vi "Main2.vi"() -> ()   [LabVIEW 2014]
doc: "This sample project is built upon the standard state machine template and shows how you could create an application that acquires, analyzes, and presents data. It includes functionality for presenting configuration dialogs, preserving settings between executions, loading and saving data, as well as exporting graph images and text files.\n\nIt is most appropriate for data that is acquired instantly as it does not allow for screen updates mid acquisition nor does it allow for continuous streaming to disk."
uses:
  controls/DAQSettings.ctl
  controls/TriggerMode.ctl
  controls/AspicSettings.ctl
  controls/AspicMode.ctl
  controls/Timeslice.ctl
  controls/SystemSet.ctl
  common/Comm/path.ctl
  controls/Data OK.ctl
  controls/Data.ctl
  controls/UI References.ctl
  controls/Graph Data.ctl
  <vilib>/Utility/miscctls.llb/LVAnnotationListTypeDef.ctl
  <vilib>/Utility/miscctls.llb/LVCursorListTypeDef.ctl
  controls/User Specified Data.ctl
  controls/HW Configuration.ctl
  controls/Simulated Signal Type.ctl
  controls/Analysis Configuration.ctl
  controls/New Data Behavior.ctl
  controls/Network.ctl
  controls/CommSelect.ctl
  common/Comm/analysis.ctl
  controls/State.ctl
  global/Global ADCarray.vi
panel:
  out "End acq":u32
  out "Begin acq":u32
  out "Path":T1={"TS file"=path "C:/Users/lpnhe/Desktop/Labview/damic/DAMIC-LTC/DamicLTC-seul-Essai.txt", "Log file"=path "C:/DAMIC/DAMIC-LTC/Data/log.txt", "Log Directory"=path "C:/DAMIC/DAMIC-LTC/Data", "Output aspic file folder"=path "C:/Users/lpnhe/Desktop/Labview/damic/DAMIC-LTC/Data", "TSfile folder"=path "C:/Users/lpnhe/Desktop/Labview/damic/DAMIC_TIMESLICE"}
  out "size(s)":i32[](array[numeric])
  in  "Curve fitting":bool
  in  "Load  Config":bool
  in  "Save  Config":bool
  in  "Path Settings":bool
  out "System Set":T2
  in  "SystemSet":bool
  in  "DAQSettings":bool
  in  "Timeslice":bool
  in  "Network Settings":bool
  in  "ASPIC Settings":bool
  in  "Snapshot":bool
  in  "Analyze":bool
  in  "Clear":bool
  in  "Exit":bool
  in  "Acquire":bool
  in  "Export":bool
  in  "Save Graph":bool
  in  "Load Graph":bool
  out "Data OK":T3
  in  "Tab Control":enum32{"Data", "Fitting", "FFT", "Results"}(tab)
  out "Time needed(s)":u32
  out "Graph":waveform(dbl)[](graph)
  in  "Display":bool
  in  "Channel":T4(ring)
  out "Results":T5
  out "timeslice":T6
  out "Aspic Seeting":T7 {"RC" format="%b"; "Gain" format="%b"}
  out "DAQ Settings":T9
  out "Status Bar":string
  # "CH0"
  # "CH1"
  # "CH2"
  # "CH3"
  # "CH4"
  # "CH5"
  # "CH6"
  # "CH7"
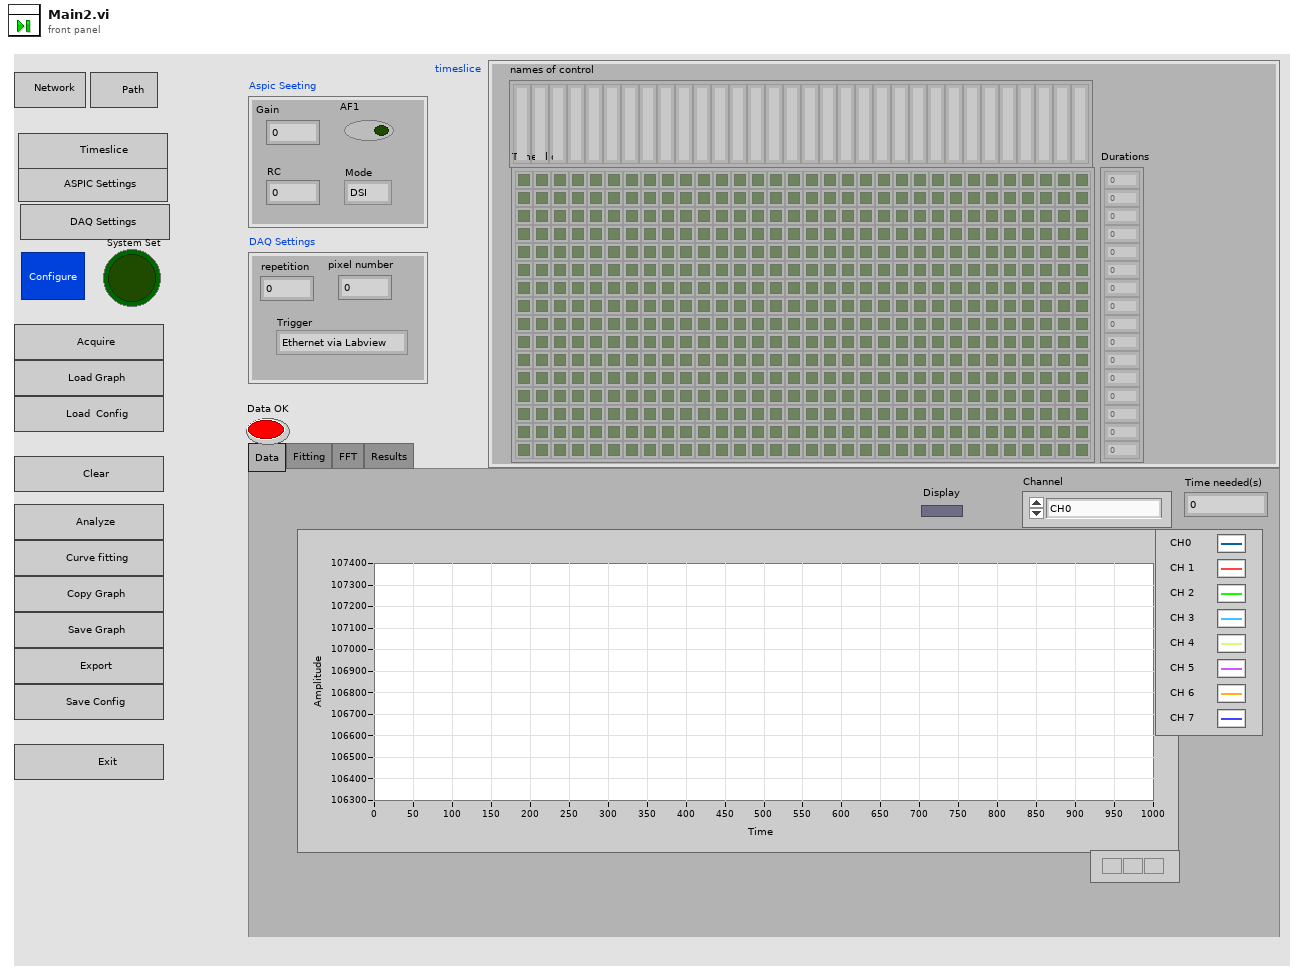
[diagram p1: front panel]
types:
  T1 = typedef "path.ctl" = cluster{"TS file":path, "Log file":path, "Log Directory":path, "Output aspic file folder":path, "TSfile folder":path}
  T2 = typedef "SystemSet.ctl" = bool
  T3 = typedef "Data OK.ctl" = bool
  T4 = enum16{"CH0", "CH1", "CH2", "CH3", "CH4", "CH5", "CH6", "CH7", "All (TDMS)"}
  T5 = cluster{"Max":i32[], "Min":i32[], "Average":dbl[], "S.D":dbl[], "Variance":dbl[]}
  T6 = typedef "Timeslice.ctl" = cluster{"Time slice":bool[][], "Durations":dbl[], "names of control":string[]}
  T7 = typedef "AspicSettings.ctl" = cluster{"Gain":u8, "RC":u8, "aspic1Data":u32[], "aspic2Data":u32[], "AF1":bool, "Mode":T8}
  T8 = typedef "AspicMode.ctl" = enum16{"DSI", "TM"}
  T9 = typedef "DAQSettings.ctl" = cluster{"pixel number":u32, "repetition":u32, "Trigger":T10}
  T10 = typedef "TriggerMode.ctl" = enum16{"Ethernet via Labview", "SMA (1.8V)"}
  T11 = typedef "State.ctl" = enum16{"Initialize", "Wait for Event", "Update UI", "Network", "Path", "Configure", "DAQSettings", "Timeslice", "Set Sytem", "Acquire", "Load Data", "Save Data", "Load config", "Save config", "Clear Data", "Export Data", "Analyze", "Curve fitting", "Copy Graph", "Exit"}
  T12 = typedef "Data.ctl" = cluster{"UI References":T13, "Graph Data":T14, "User Specified":T17, "System Set":T2, "Results":T24, "Data OK":T3}
  T13 = typedef "UI References.ctl" = cluster{"Exit Ref":refnum<vi>, "Save Ref":refnum<vi>, "Open Ref":refnum<vi>, "Export Ref":refnum<vi>, "Acquire Ref":refnum<vi>, "Configure Ref":refnum<vi>, "Graph Ref":refnum<vi>, "Clear Ref":refnum<vi>, "Analyze Ref":refnum<vi>, "Status Ref":refnum<vi>, "Snapshot Ref":refnum<vi>, "Network Ref":refnum<vi>, "Timeslice Ref":refnum<vi>, "DAQSetting Ref":refnum<vi>, "SystemSet":refnum<vi>, "Path ref":refnum<vi>, "Data OK Ref":refnum<vi>}
  T14 = typedef "Graph Data.ctl" = cluster{"Data":waveform(dbl)[], "Annotation List":T15, "Cursor List":T16, "Analysis Data":waveform(dbl)[]}
  T15 = typedef "LVAnnotationListTypeDef.ctl" = cluster{"Name":string, "Color":u32, "Style":u8, "Point Style":u8, "Name Visible":bool, "Allow Drag":bool, "Annotation Mode":u32, "Plot":i32, "Index":i32, "Position":cluster{"X":dbl, "Y":dbl}, "X Scale":u32, "Y Scale":u32, "Show Arrow":bool, "Lock Name":bool, "Plot Area":i32, "Label Offset":cluster{"X":dbl, "Y":dbl}}[]
  T16 = typedef "LVCursorListTypeDef.ctl" = cluster{"Name":string, "Color":u32, "Style":u8, "Point Style":u8, "Name Visible":bool, "Allow Drag":bool, "Cursor Mode":u32, "Plot":i32, "Index":i32, "Position":cluster{"X":dbl, "Y":dbl}, "X Scale":u32, "Y Scale":u32, "Watch Plots":i32[], "Watch All Plots":bool, "Plot Area":i32, "Label Offset":cluster{"X":dbl, "Y":dbl}}[]
  T17 = typedef "User Specified Data.ctl" = cluster{"Hardware Configuration":T18, "Analysis Configuration":T20, "New Data Behavior":T21, "Aspic Seeting":T7, "Network":T22, "timeslice":T6, "Acquisition Settings":T9, "CommSelect":T23, "Path":T1}
  T18 = typedef "HW Configuration.ctl" = cluster{"HW Refnum <Replace Me>":string, "Signal Type <Replace Me>":T19}
  T19 = typedef "Simulated Signal Type.ctl" = enum16{"Sine Wave", "Square Wave"}
  T20 = typedef "Analysis Configuration.ctl" = cluster{"Statistics":bool}
  T21 = typedef "New Data Behavior.ctl" = enum16{"Replace", "Overlay", "Append"}
  T22 = typedef "Network.ctl" = cluster{"invert_send":bool, "Number of datagrams to read":u32, "max bytes/read":i32, "Timeout":i32, "host":string, "Port Receive":u16}
  T23 = typedef "CommSelect.ctl" = enum16{"startTSL", "writeCABAC", "readCABAC", "resetCABAC", "emissionTest", "regRead", "executeASPIC", "resetASPIC", "resetFifo18ASPIC", "resetFifo16ASPIC", "LabviewDamicStart"}
  T24 = typedef "analysis.ctl" = cluster{"Max":i32[], "Min":i32[], "Average":dbl[], "S.D":dbl[], "Variance":dbl[]}
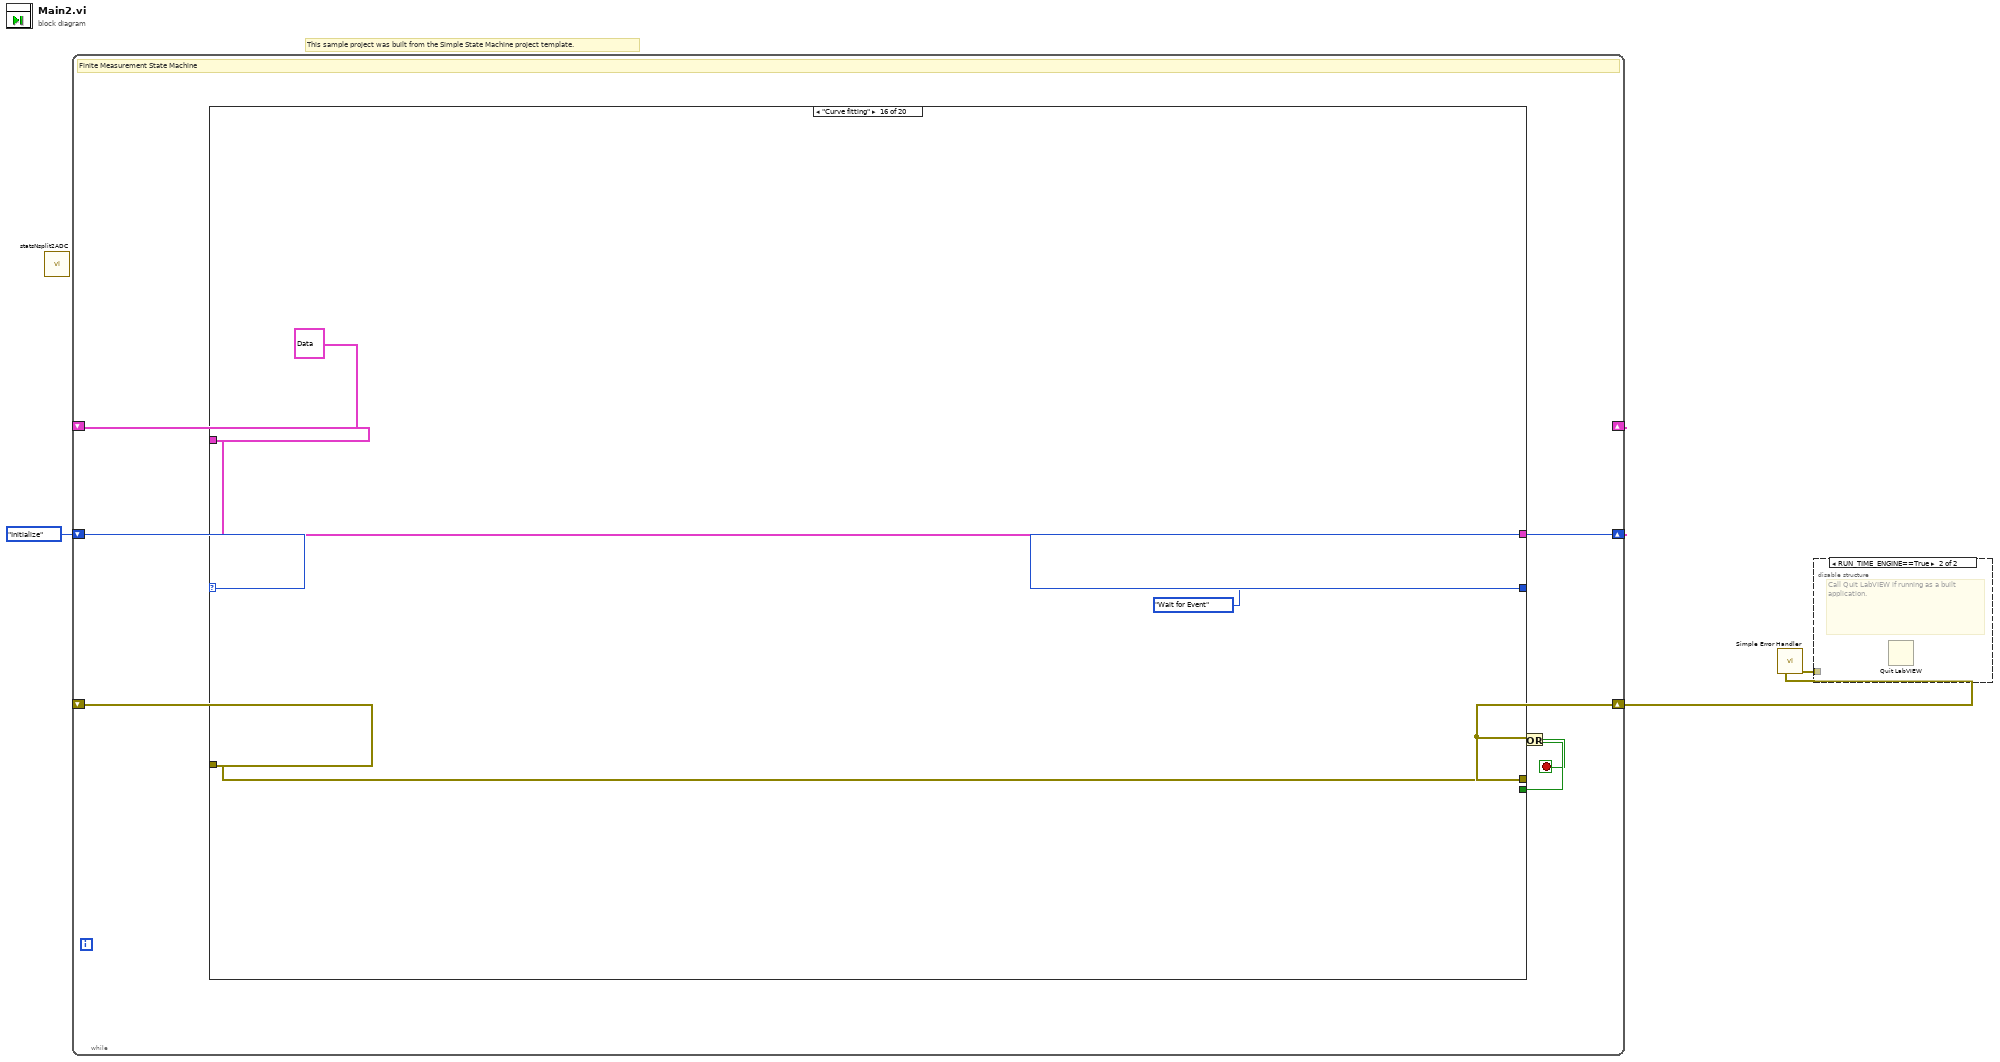
[diagram p0: block diagram]
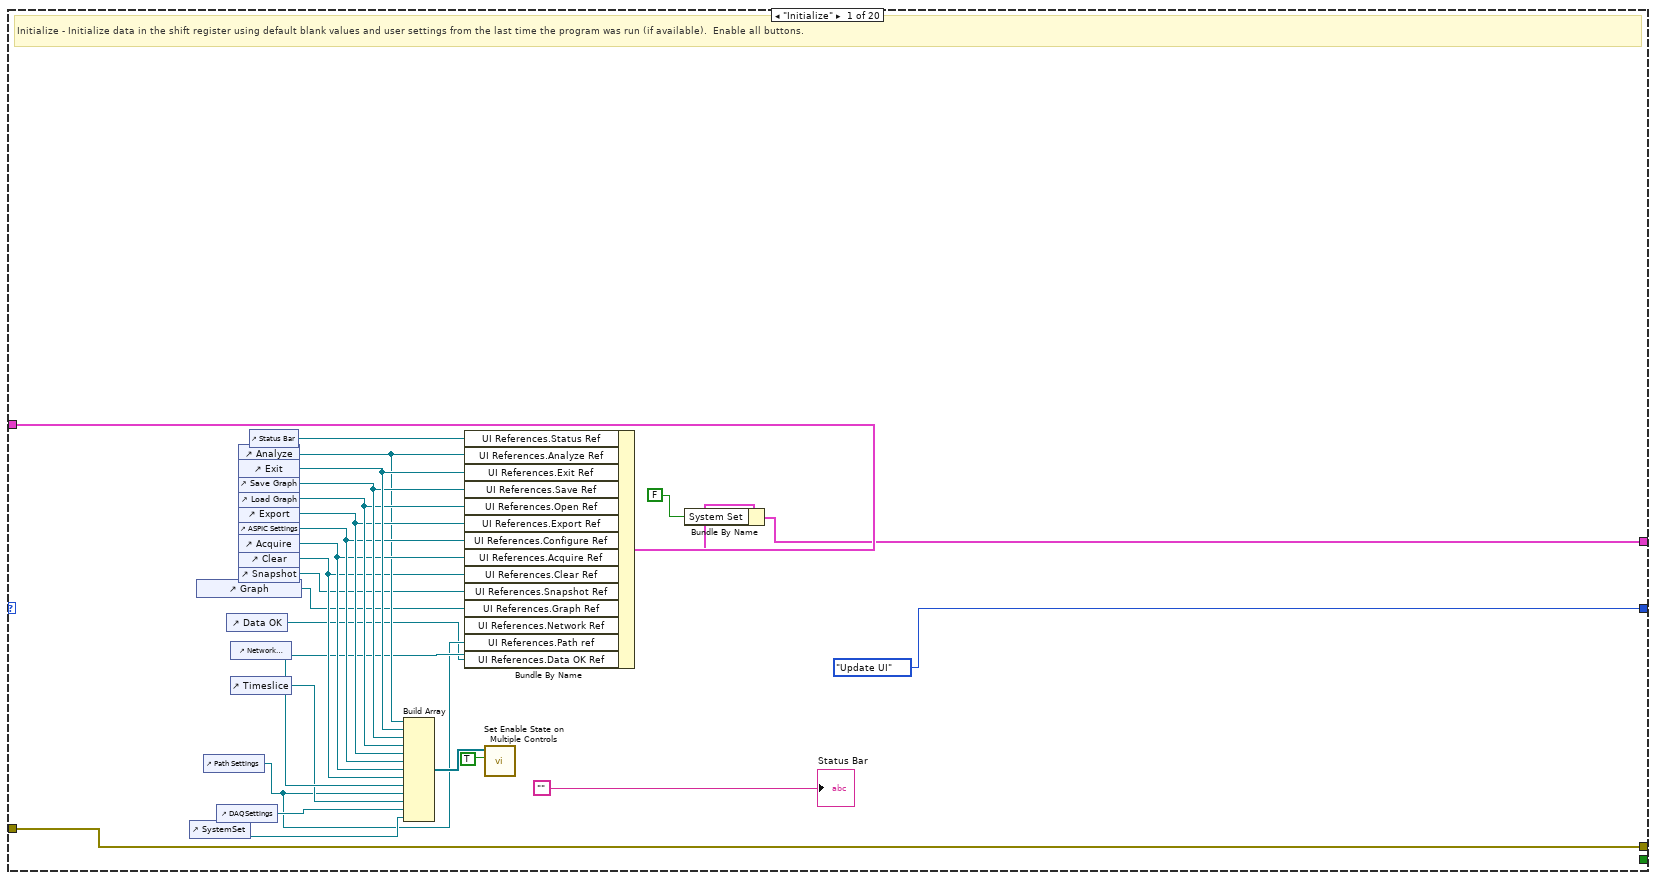
[diagram p3: hidden frame]
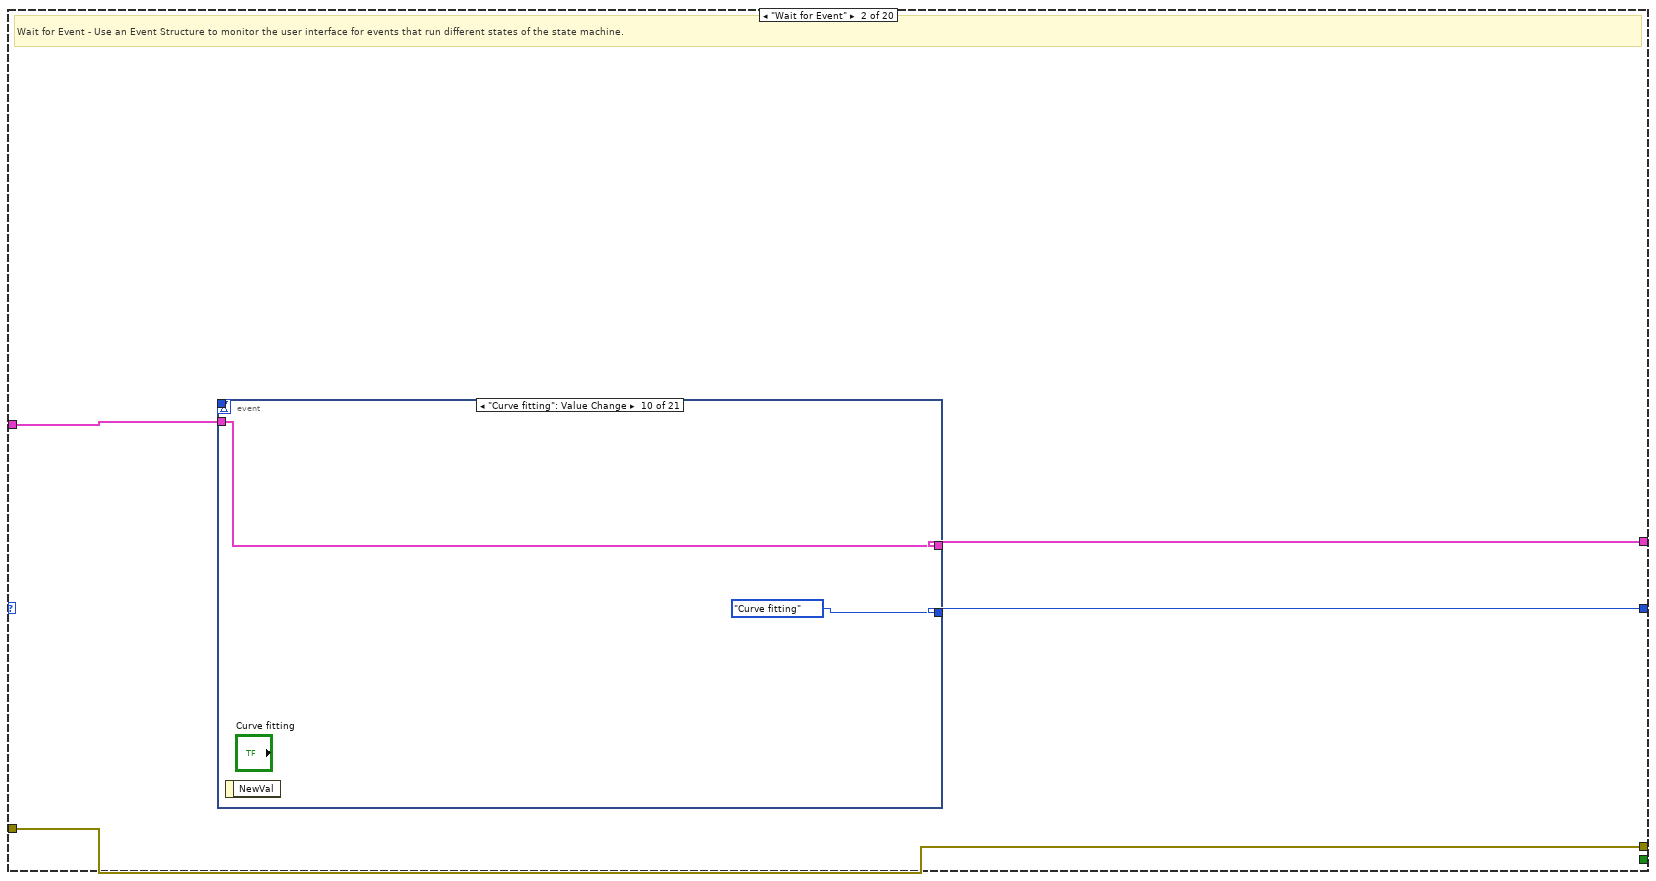
[diagram p4: hidden frame]
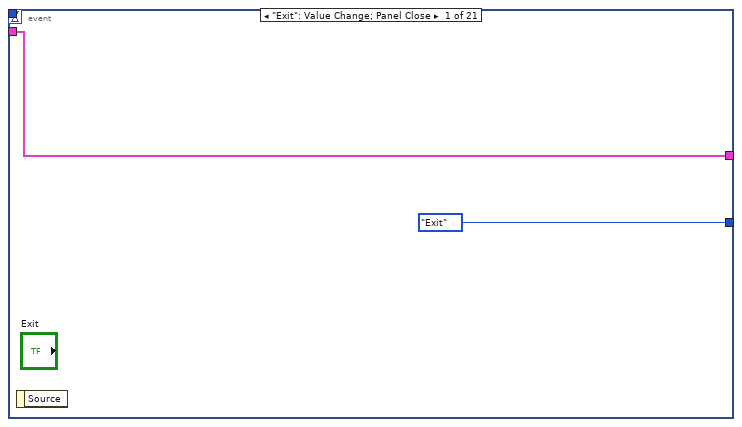
[diagram p5: hidden frame]
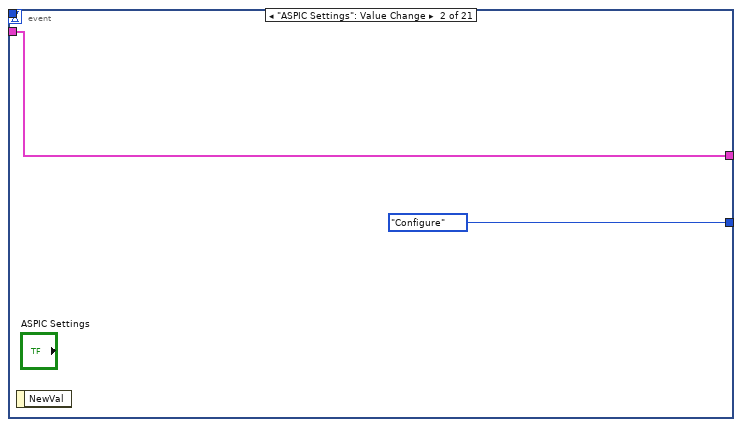
[diagram p6: hidden frame]
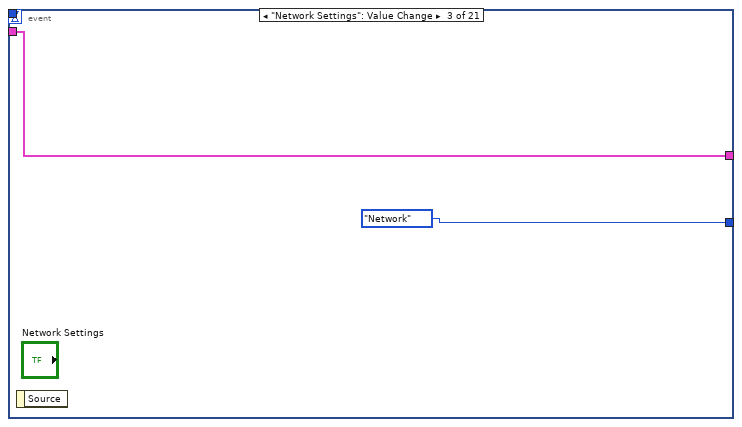
[diagram p7: hidden frame]
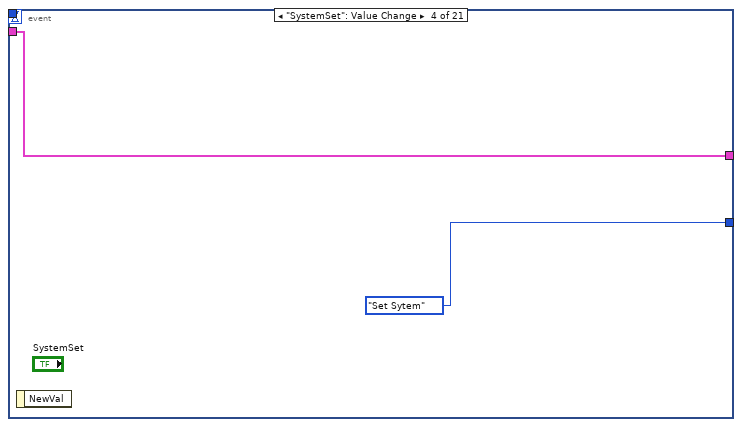
[diagram p8: hidden frame]
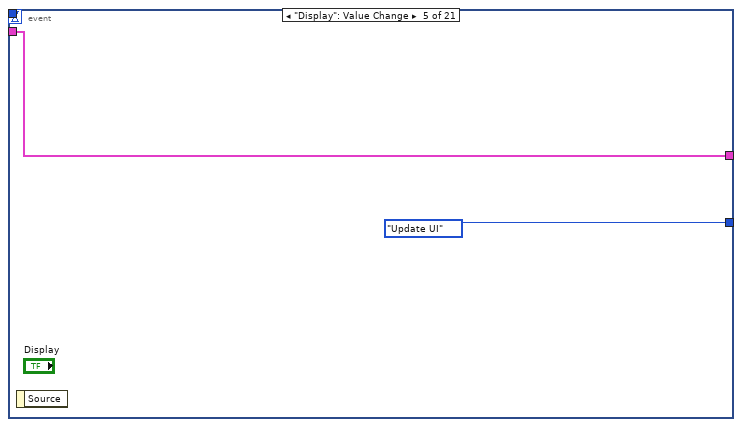
[diagram p9: hidden frame]
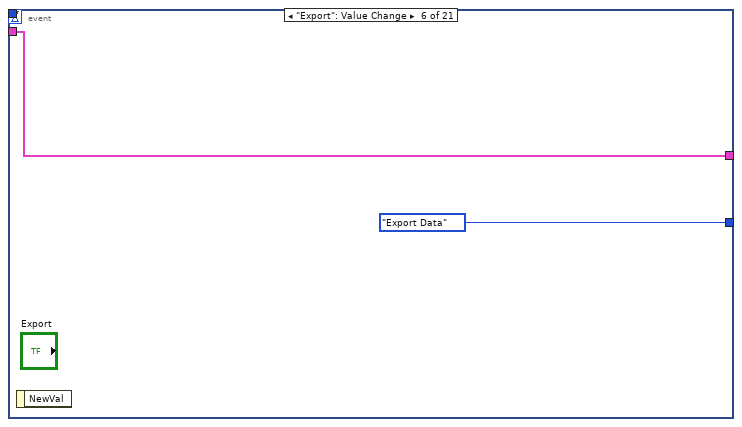
[diagram p10: hidden frame]
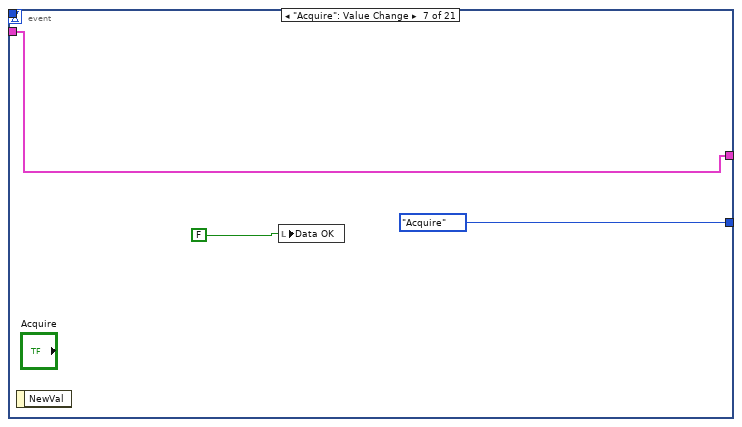
[diagram p11: hidden frame]
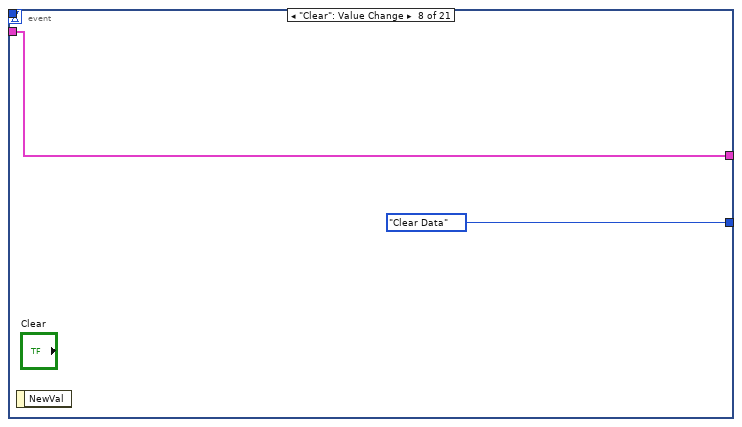
[diagram p12: hidden frame]
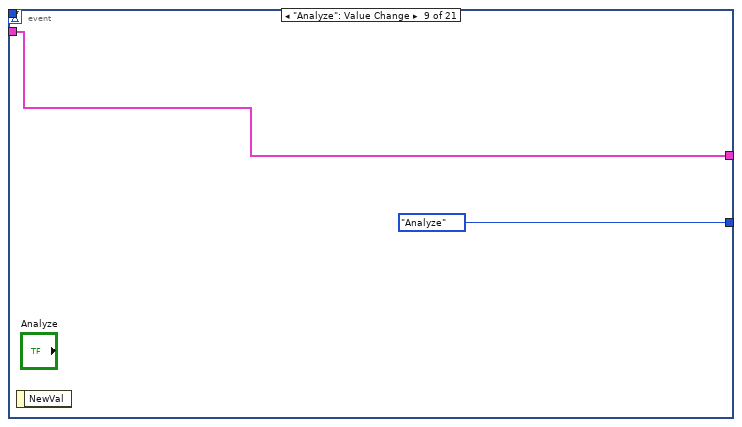
[diagram p13: hidden frame]
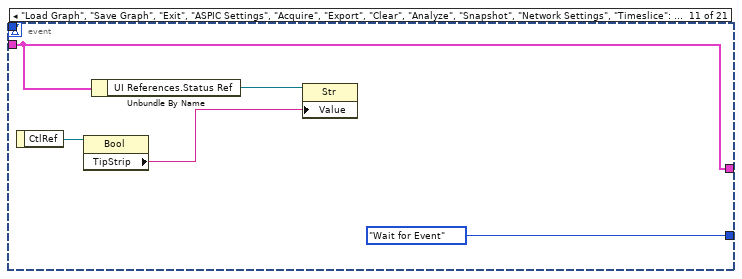
[diagram p14: hidden frame]
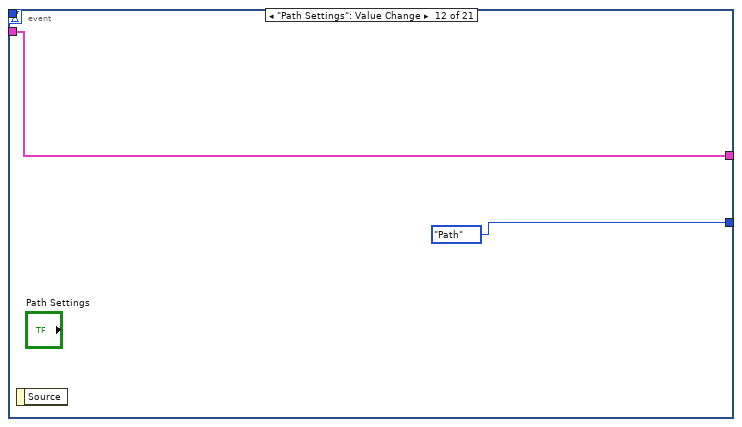
[diagram p15: hidden frame]
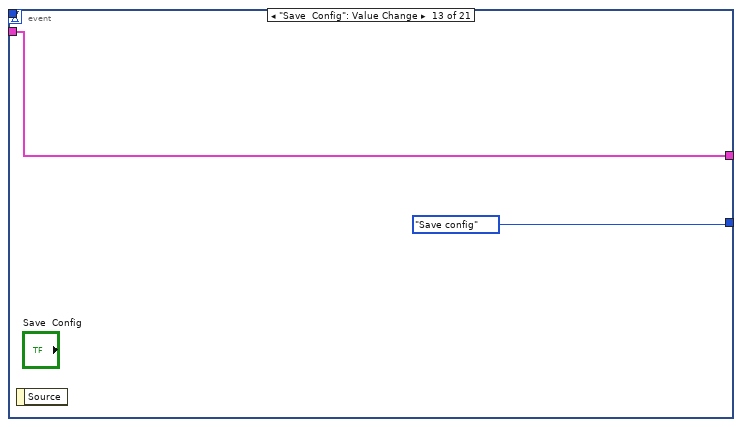
[diagram p16: hidden frame]
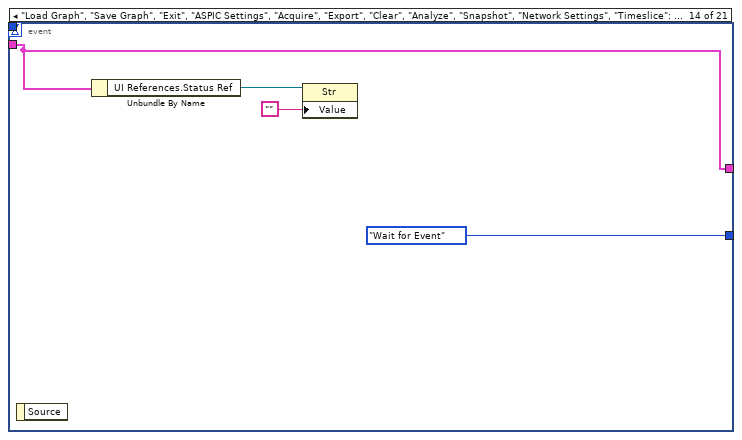
[diagram p17: hidden frame]
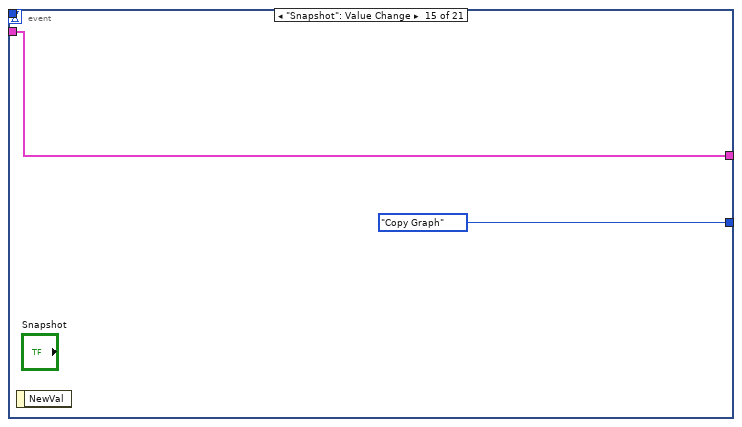
[diagram p18: hidden frame]
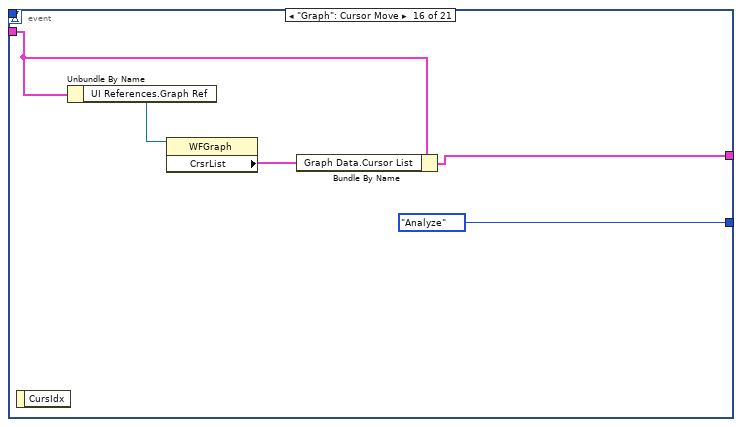
[diagram p19: hidden frame]
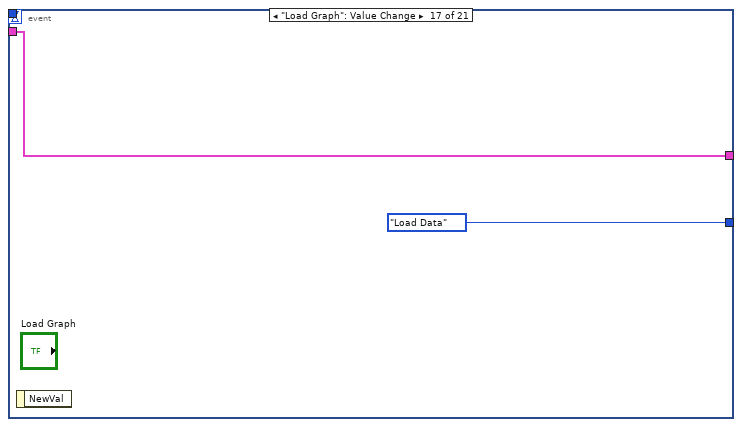
[diagram p20: hidden frame]
diagram:
  # "This sample project was built from the Simple State Machine project template."
  n1 = call "statsNsplit2ADC.vi"() -> ()  [unwired: 4 in, 4 out]
  n2 = while {
    shift-right: [w11] -> _
    shift-left: State."Initialize" ("Next State") -> [w12]
    shift-right: [w5] -> w4
    shift-left: _ -> [w6]
    shift-right: [w7] -> _
    shift-left: T12 {"UI References"={"Exit Ref"=refnum, "Save Ref"=refnum, "Open Ref"=refnum, "Export Ref"=refnum, "Acquire Ref"=refnum, "Configure Ref"=refnum, "Graph Ref"=refnum, "Clear Ref"=refnum, "Analyze Ref"=refnum, "Status Ref"=refnum, "Snapshot Ref"=refnum, "Network Ref"=refnum, "Timeslice Ref"=refnum, "DAQSetting Ref"=refnum, "SystemSet"=refnum, "Path ref"=refnum, "Data OK Ref"=refnum}, "Graph Data"={"Data"=[], "Annotation List"=[], "Cursor List"=[], "Analysis Data"=[]}, "User Specified"={"Hardware Configuration"={"HW Refnum <Replace Me>"="", "Signal Type <Replace Me>"=enum."Sine Wave"}, "Analysis Configuration"={"Statistics"=TRUE}, "New Data Behavior"=enum."Replace", "Aspic Seeting"={"Gain"=0, "RC"=0, "aspic1Data"=[], "aspic2Data"=[], "AF1"=FALSE, "Mode"=enum."TM"}, "Network"={"invert_send"=TRUE, "Number of datagrams to read"=5000, "max bytes/read"=2500, "Timeout"=4000, "host"="192.168.1.18", "Port Receive"=5678}, "timeslice"={"Time slice"=[], "Durations"=[], "names of control"=[]}, "Acquisition Settings"={"pixel number"=0, "repetition"=0, "Trigger"=enum."Ethernet via Labview"}, "CommSelect"=enum."resetFifo18ASPIC", "Path"={"TS file"=path "C:/Users/lpnhe/Desktop/Labview/damic/DAMIC-LTC/DamicLTC-seul-Essai.txt", "Log file"=path "C:/DAMIC/DAMIC-LTC/Data/log.txt", "Log Directory"=path "C:/DAMIC/DAMIC-LTC/Data", "Output aspic file folder"=path "C:/Users/lpnhe/Desktop/Labview/damic/DAMIC-LTC/Data", "TSfile folder"=path "C:/Users/lpnhe/Desktop/Labview/damic/DAMIC_TIMESLICE"}}, "System Set"=FALSE, "Results"={"Max"=[], "Min"=[], "Average"=[], "S.D"=[], "Variance"=[]}, "Data OK"=FALSE} ("Data") -> [w8]
    stop <- w9 stop-if-true
    # "Finite Measurement State Machine"
    n3 = case shown="\"Curve fitting\"" w12 {
      tunnel: [State."Update UI" ("Next State") w42 State."Wait for Event" ("(Value Not Used)") State."Update UI" ("Next State if true") w154 State."Update UI" ("Next State if true") State."Update UI" ("Next State if true") w184 State."Update UI" ("States") w230 State."Update UI" ("(Value Not Used)") State."Wait for Event" ("(Value Not Used)") State."Wait for Event" ("(Value Not Used)") State."Update UI" ("(Value Not Used)") State."Update UI" ("(Value Not Used)") State."Wait for Event" ("Next State") State."Wait for Event" ("(Value Not Used)") w338 State."Update UI" ("Next State") State."Wait for Event" ("Next State")] -> w11
      tunnel: [_ _ _ _ _ _ _ _ _ _ _ _ _ _ _ _ _ w337 _ _] -> w10
      tunnel: w8 -> [w17 w41 w105 w144 w155 w166 w173 w182 w198 w229 w276 w292 w305 w318 w323 w329 w333 w336 w344 w349]
      tunnel: [w14 w40 w105 w138 w146 w158 w167 w176 w194 w226 w275 w292 w305 w317 w321 w329 w333 w336 w343 w349] -> w7
      tunnel: w6 -> [w22 w39 w106 w142 w152 w165 w172 w188 w196 w228 w273 w291 w304 w316 w325 w328 w332 w335 w341 w351]
      tunnel: [w22 w39 w106 w141 w151 w162 w171 w188 w189 w227 w272 w290 w303 w316 w324 w328 w331 w335 w340 w350] -> w5
      frame "Initialize" {
        # "Initialize - Initialize data in the shift register using default blank values and user settings from the last time the program was run (if available).  Enable all buttons."
        n4 = control-ref of="SystemSet"() -> (w19:refnum<vi>)
        n5 = control-ref of="Graph"() -> (w24:refnum<vi>)
        n6 = control-ref of="Path Settings"() -> (w18:refnum<vi>)
        n7 = control-ref of="DAQSettings"() -> (w20:refnum<vi>)
        n8 = control-ref of="Data OK"() -> (w13:refnum<vi>)
        n9 = control-ref of="Network Settings"() -> (w23:refnum<vi>)
        n10 = control-ref of="Timeslice"() -> (w21:refnum<vi>)
        n11 = control-ref of="Analyze"() -> (w30:refnum<vi>)
        n12 = control-ref of="Exit"() -> (w37:refnum<vi>)
        n13 = control-ref of="Save Graph"() -> (w36:refnum<vi>)
        n14 = control-ref of="Load Graph"() -> (w35:refnum<vi>)
        n15 = control-ref of="Export"() -> (w34:refnum<vi>)
        n16 = control-ref of="ASPIC Settings"() -> (w33:refnum<vi>)
        n17 = control-ref of="Acquire"() -> (w32:refnum<vi>)
        n18 = control-ref of="Clear"() -> (w28:refnum<vi>)
        n19 = control-ref of="Snapshot"() -> (w25:refnum<vi>)
        n20 = control-ref of="Status Bar"() -> (w29:refnum<vi>)
        n21 = Build Array(w30, w37, w36, w35, w34, w33, w32, w28, w23, w18, w21, w20, w19) -> (w31:refnum<vi>[])
        n22 = Bundle By Name(cluster=w17, "UI References.Status Ref"=w29, "UI References.Analyze Ref"=w30, "UI References.Exit Ref"=w37, "UI References.Save Ref"=w36, "UI References.Open Ref"=w35, "UI References.Export Ref"=w34, "UI References.Configure Ref"=w33, "UI References.Acquire Ref"=w32, "UI References.Clear Ref"=w28, "UI References.Snapshot Ref"=w25, "UI References.Graph Ref"=w24, "UI References.Network Ref"=w23, "UI References.Path ref"=w18, "UI References.Data OK Ref"=w13) -> (w16:T12)
        n23 = call "Set Enable State on Multiple Controls.vi"("Enable?"=TRUE, "Controls"=w31) -> ()  [unwired: 10 in]
        n24 = Bundle By Name(cluster=w16, "System Set"=FALSE) -> (w14:T12)
        "Status Bar" <- "" ("Status Bar")
      }
      frame "Wait for Event" {
        # "Wait for Event - Use an Event Structure to monitor the user interface for events that run different states of the state machine."
        n25 = event shown="[9] \"Curve fitting\": Value Change" {
          selector: _ -> [_ _ _ _ _ _ _ _ _ _ _ _ _ _ _ _ _ _ _ _ _]
          dyn-events: _ -> [_ _ _ _ _ _ _ _ _ _ _ _ _ _ _ _ _ _ _ _ _]
          timeout: _ -> [_ w46 _ _ _ _ _ _ _ _ _ _ _ _ _ _ _ _ _ _ _]
          tunnel: [State."Exit" ("Next State") State."Configure" ("Next State") State."Network" ("States") State."Set Sytem" ("States") State."Update UI" ("States") State."Export Data" ("Next State") State."Acquire" ("Next State") State."Clear Data" ("Next State") State."Analyze" ("Next State") State."Curve fitting" ("Next State") State."Wait for Event" ("Next State") State."Path" ("Next State") State."Save config" ("Next State") State."Wait for Event" ("Next State") State."Copy Graph" ("Next State") State."Analyze" ("Next State") State."Load Data" ("Next State") State."Save Data" ("Next State") State."Load config" ("Next State") State."Timeslice" ("States") State."DAQSettings" ("States")] -> w42
          tunnel: [_ w46 _ _ _ _ _ _ _ _ _ _ _ _ _ _ _ _ _ _ _] -> _
          tunnel: w41 -> [w43 w45 w49 w51 w53 w54 w57 w59 w61 w64 w65 w71 w73 w74 w78 w81 w85 w87 w90 w92 w94]
          tunnel: [w43 w45 w49 w51 w53 w54 w57 w59 w61 w64 w65 w71 w73 w74 w78 w80 w85 w87 w90 w92 w94] -> w40
          event "Exit": Value Change; Panel Close {
            n26 = event-data() -> ()  [unwired: 1 in, 1 out]
          }
          event "ASPIC Settings": Value Change {
            n27 = event-data() -> ()  [unwired: 1 in, 1 out]
          }
          event "Network Settings": Value Change {
            n28 = event-data() -> ()  [unwired: 1 in, 1 out]
          }
          event "SystemSet": Value Change {
            n29 = event-data() -> ()  [unwired: 1 in, 1 out]
          }
          event "Display": Value Change {
            n30 = event-data() -> ()  [unwired: 1 in, 1 out]
          }
          event "Export": Value Change {
            n31 = event-data() -> ()  [unwired: 1 in, 1 out]
          }
          event "Acquire": Value Change {
            n32 = event-data() -> ()  [unwired: 1 in, 1 out]
            n33 = local write "Data OK"(FALSE) -> ()
          }
          event "Clear": Value Change {
            n34 = event-data() -> ()  [unwired: 1 in, 1 out]
          }
          event "Analyze": Value Change {
            n35 = event-data() -> ()  [unwired: 1 in, 1 out]
          }
          event "Curve fitting": Value Change {
            n36 = event-data() -> ()  [unwired: 1 in, 1 out]
          }
          event "Load Graph", "Save Graph", "Exit", "ASPIC Settings", "Acquire", "Export", "Clear", "Analyze", "Snapshot", "Network Settings", "Timeslice": Mouse Enter {
            n37 = event-data() -> ("CtlRef"=w69:refnum<vi>)  [unwired: 1 in]
            n38 = property class="Bool"(reference=w69) -> ("TipStrip"=w67:string)  [unwired: 1 in, 2 out]
            n39 = Unbundle By Name(w65) -> ("UI References.Status Ref"=w68:refnum<vi>)
            n40 = property class="Str"(reference=w68, "Value"=w67) -> ()  [unwired: 1 in, 2 out]
          }
          event "Path Settings": Value Change {
            n41 = event-data() -> ()  [unwired: 1 in, 1 out]
          }
          event "Save  Config": Value Change {
            n42 = event-data() -> ()  [unwired: 1 in, 1 out]
          }
          event "Load Graph", "Save Graph", "Exit", "ASPIC Settings", "Acquire", "Export", "Clear", "Analyze", "Snapshot", "Network Settings", "Timeslice": Mouse Leave {
            n43 = event-data() -> ()  [unwired: 1 in, 1 out]
            n44 = Unbundle By Name(w74) -> ("UI References.Status Ref"=w77:refnum<vi>)
            n45 = property class="Str"(reference=w77, "Value"="") -> ()  [unwired: 1 in, 2 out]
          }
          event "Snapshot": Value Change {
            n46 = event-data() -> ()  [unwired: 1 in, 1 out]
          }
          event "Graph": Cursor Move {
            n47 = event-data() -> ()  [unwired: 1 in, 1 out]
            n48 = Unbundle By Name(w81) -> ("UI References.Graph Ref"=w83:refnum<vi>)
            n49 = property class="WFGraph"(reference=w83) -> ("CrsrList"=w82:T16)  [unwired: 1 in, 2 out]
            n50 = Bundle By Name(cluster=w81, "Graph Data.Cursor List"=w82) -> (w80:T12)
          }
          event "Load Graph": Value Change {
            n51 = event-data() -> ()  [unwired: 1 in, 1 out]
          }
          event "Save Graph": Value Change {
            n52 = event-data() -> ()  [unwired: 1 in, 1 out]
          }
          event "Load  Config": Value Change {
            n53 = event-data() -> ()  [unwired: 1 in, 1 out]
          }
          event "Timeslice": Value Change {
            n54 = event-data() -> ()  [unwired: 1 in, 1 out]
          }
          event "DAQSettings": Value Change {
            n55 = event-data() -> ()  [unwired: 1 in, 1 out]
          }
        }
      }
      frame "Update UI" {
        # "These buttons should be disabled when there is no data visible."
        # "Update UI - Update the graph using the waveform data stored in the shift register.  If there is no data to display disable buttons that act on the current data."
        n56 = Unbundle By Name(w105) -> ("Results"=→"Results":T24, "Graph Data.Data"=w99:waveform(dbl)[], "Graph Data.Annotation List"=w109:T15, "Graph Data.Cursor List"=w108:T16)
        n57 = Unbundle By Name(w105) -> ("User Specified.Path"=→"Path":T1, "User Specified.timeslice"=→"timeslice":T6, "User Specified.Aspic Seeting"=→"Aspic Seeting":T7, "User Specified.Acquisition Settings"=→"DAQ Settings":T9, "System Set"=→"System Set":T2, "Data OK"=→"Data OK":T3)
        n58 = Unbundle By Name(w105) -> ("UI References.Clear Ref"=w115:refnum<vi>, "UI References.Analyze Ref"=w114:refnum<vi>, "UI References.Save Ref"=w118:refnum<vi>, "UI References.Export Ref"=w112:refnum<vi>, "UI References.Snapshot Ref"=w113:refnum<vi>)
        n59 = case shown="\"All (TDMS)\"" "Channel" {
          tunnel: w99 -> [w121 w123 w125 w127 w129 w131 w133 w135 w136]
          tunnel: [w120 w122 w124 w126 w128 w130 w132 w134 w136] -> w98
          frame "CH0", Default {
            n60 = Decimate 1D Array(w121) -> (w120:waveform(dbl)[])  [unwired: 7 out]
          }
          frame "CH1" {
            n61 = Decimate 1D Array(w123) -> (w122:waveform(dbl)[])  [unwired: 7 out]
          }
          frame "CH2" {
            n62 = Decimate 1D Array(w125) -> (w124:waveform(dbl)[])  [unwired: 7 out]
          }
          frame "CH3" {
            n63 = Decimate 1D Array(w127) -> (w126:waveform(dbl)[])  [unwired: 7 out]
          }
          frame "CH4" {
            n64 = Decimate 1D Array(w129) -> (w128:waveform(dbl)[])  [unwired: 7 out]
          }
          frame "CH5" {
            n65 = Decimate 1D Array(w131) -> (w130:waveform(dbl)[])  [unwired: 7 out]
          }
          frame "CH6" {
            n66 = Decimate 1D Array(w133) -> (w132:waveform(dbl)[])  [unwired: 7 out]
          }
          frame "CH7" {
            n67 = Decimate 1D Array(w135) -> (w134:waveform(dbl)[])  [unwired: 7 out]
          }
          frame "All (TDMS)" {
          }
        }
        "Graph" <- w98
        n68 = Array Size(array=w99) -> (size(s)=w117:i32)
        n69 = Not Equal To 0?(x=w117) -> (x != 0?=w116:bool)
        n70 = call "Get Scale Labels.vi"("Array of Waveforms"=w99) -> ("Y Scale Label Text"=w110:string, "X Scale Label Text"=w111:string)  [unwired: 9 in]
        n71 = Build Array(w115, w114, w118, w112, w113) -> (w107:refnum<vi>[])
        n72 = property on="Graph" class="WFGraph (strict)"("AnntList"=w109, "CrsrList"=w108, "LegNumRows"=w117, "XScale.NameLbl.Text"=w111, "YScale.NameLbl.Text"=w110) -> ()  [unwired: 2 in, 2 out]
        n73 = call "Set Enable State on Multiple Controls.vi"("Enable?"=w116, "Controls"=w107) -> ()  [unwired: 10 in]
      }
      frame "Network" {
        n74 = Unbundle By Name(w144) -> ("User Specified.Network"=w145:T22)
        n75 = call "NetworkSettingsDialog.vi"("error in (no error)"=w142, "Network In"=w145) -> ("error out"=w141:errorcluster, "Network Out"=w143:T22)  [unwired: 7 in, 1 out]
        n76 = Bundle By Name(cluster=w144, "User Specified.Network"=w143) -> (w140:T12)
        n77 = Bundle By Name(cluster=w140, "System Set"=FALSE) -> (w138:T12)
      }
      frame "Path" {
        n78 = Unbundle By Name(w155) -> ("User Specified.Path"=w153:T1)
        n79 = call "PathSettingDialog.vi"("Path in"=w153, "error in (no error)"=w152) -> ("Path out"=w149:T1, "UI Refresh Needed ?"=w150:bool, "error out"=w151:errorcluster)  [unwired: 15 in]
        n80 = Select(t=State."Update UI" ("Next State if true"), s=w150, f=State."Wait for Event" ("Next State if faut")) -> (s? t:f=w154:T11)
        n81 = Bundle By Name(cluster=w155, "User Specified.Path"=w149) -> (w148:T12)
        n82 = Bundle By Name(cluster=w148, "System Set"=FALSE) -> (w146:T12)
      }
      frame "Configure" {
        # "Configure - Spawns a dialog that allows the user to set any user configurable settings."
        n83 = Unbundle By Name(w166) -> ("User Specified.Aspic Seeting"=w164:T7)
        n84 = call "AspicSettingsDialog.vi"("error in (no error)"=w165, "Aspic Seeting In"=w164) -> ("error out"=w162:errorcluster, "Aspic Seeting Out"=w163:T7)  [unwired: 5 in, 1 out]
        n85 = Bundle By Name(cluster=w166, "User Specified.Aspic Seeting"=w163) -> (w159:T12)
        n86 = Bundle By Name(cluster=w159, "System Set"=FALSE) -> (w158:T12)
      }
      frame "DAQSettings" {
        n87 = Unbundle By Name(w173) -> ("User Specified.Acquisition Settings"=w175:T9)
        n88 = call "DAQSettingsDialog.vi"("error in (no error)"=w172, "Acquisition Settings In"=w175) -> ("error out"=w171:errorcluster, "Acquisition Settings Out"=w174:T9)  [unwired: 7 in, 1 out]
        n89 = Bundle By Name(cluster=w173, "User Specified.Acquisition Settings"=w174) -> (w168:T12)
        n90 = Bundle By Name(cluster=w168, "System Set"=FALSE) -> (w167:T12)
      }
      frame "Timeslice" {
        n91 = Unbundle By Name(w182) -> ("User Specified.timeslice"=w183:T6)
        n92 = call "SetTimesliceDialog.vi"("timeslice in"=w183) -> ("timeslice out"=w181:T6)  [unwired: 10 in]
        n93 = Bundle By Name(cluster=w182, "User Specified.timeslice"=w181) -> (w177:T12)
        n94 = Unbundle By Name(w177) -> ("User Specified.timeslice.Time slice"=w180:bool[][])
        n95 = Array Size(array=w180) -> (size(s)=→"size(s)":i32[])
        n96 = Select(t=State."Update UI" ("Next State if true"), s=TRUE, f=State."Wait for Event" ("Next State if false")) -> (s? t:f=w184:T11)
        n97 = Bundle By Name(cluster=w177, "System Set"=FALSE) -> (w176:T12)
      }
      frame "Set Sytem" {
        # "reset the FIFO of the FPGA"
        # "ASPIC gain / RC etc"
        n98 = flat-sequence {
          tunnel: w198 -> [w203]
          tunnel: [w201] -> w197
          tunnel: w196 -> [_]
          tunnel: [w200] -> w195
          tunnel: w197 -> [w210]
          tunnel: w195 -> [w209]
          tunnel: [w210] -> w192
          tunnel: [w205] -> w190
          tunnel: w192 -> [w212]
          tunnel: [w212] -> w191
          tunnel: w190 -> [w211]
          tunnel: [w211] -> w189
          tunnel: [w215] -> w194
          tunnel: w191 -> [w217]
          frame #0 {
            n99 = Unbundle By Name(w203) -> ("User Specified.Aspic Seeting"=w204:T7, "User Specified.Acquisition Settings"=w199:T9)
            n100 = call "SetASPIC.vi"("Acquisition Settings"=w199, "Aspic Seeting In"=w204) -> ("error out"=w200:errorcluster, "Aspic Seeting Out"=w202:T7)  [unwired: 8 in]
            n101 = Bundle By Name(cluster=w203, "User Specified.Aspic Seeting"=w202) -> (w201:T12)
          }
          frame #1 {
            n102 = call "programComm.vi"("error in (no error)"=w209, "CommSelect"=CommSelect."resetFifo16ASPIC") -> ("error out"=w206:errorcluster)
            n103 = call "programComm.vi"("error in (no error)"=w206, "CommSelect"=CommSelect."resetFifo18ASPIC") -> ("error out"=w205:errorcluster)
          }
          frame #2 {
            n104 = Unbundle By Name(w212) -> ("User Specified.timeslice"=w214:T6, "User Specified.Acquisition Settings"=w213:T9)
            n105 = call "SetTS.vi"("Acquisition Settings"=w213, "timeslice"=w214) -> ()  [unwired: 10 in]
          }
          frame #3 {
            n106 = Bundle By Name(cluster=w217, "System Set"=TRUE) -> (w215:T12)
          }
        }
      }
      frame "Acquire" {
        # "Acquire - Uses the current hardware configuration to acquire a new data set and stores it in the state data."
        n107 = flat-sequence {
          tunnel: w228 -> [w232]
          tunnel: w229 -> [w233]
          tunnel: [w233] -> w225
          tunnel: [w232] -> w224
          tunnel: w225 -> [w243]
          tunnel: w224 -> [w242]
          tunnel: [State."Update UI" ("Next State")] -> w223
          tunnel: [w241] -> w222
          tunnel: [w236] -> w221
          tunnel: w223 -> [w263]
          tunnel: w222 -> [w262]
          tunnel: w221 -> [w261]
          tunnel: [w263] -> w220
          tunnel: [w262] -> w219
          tunnel: [w261] -> w218
          tunnel: [w269] -> w226
          tunnel: [w270] -> w227
          tunnel: [w271] -> w230
          tunnel: w220 -> [w271]
          tunnel: w219 -> [w270]
          tunnel: w218 -> [w269]
          frame #0 {
            n108 = Tick Count (ms)() -> (millisecond timer value=→"Begin acq":u32)
          }
          frame #1 {
            n109 = Unbundle By Name(w243) -> ("UI References.Status Ref"=w244:refnum<vi>, "User Specified.Acquisition Settings"=w248:T9, "User Specified.Network"=w240:T22)
            n110 = call "Acquire Data from Hardware.vi"("error in (no error)"=w242, "read"=TRUE, "Network"=w240, "Acquisition Settings"=w248) -> ("error out"=w245:errorcluster, "Graph Data 2"=w237:T14, "Graph Data"=w246:waveform(dbl)[])  [unwired: 5 in]
            n111 = case shown="No Error" w245 {
              selector: w245 -> [w253 w259]
              tunnel: [w255 w257] -> w238
              tunnel: w246 -> [w254 _]
              tunnel: ["Data acquired." ("Data acquired") "Data not acquired." ("Data not acquired")] -> w247
              tunnel: w243 -> [w251 w257]
              tunnel: [w250 w256] -> w241
              frame No Error {
                n112 = call "Incorporate New Data.vi"("error in (no error)"=w253, "New Graph Data"=w254, "Data in"=w251) -> ("error out"=w250:errorcluster, "Data out"=w255:T12)  [unwired: 7 in]
              }
              frame Error {
                n113 = call <vilib>:"Simple Error Handler.vi"("error in (no error)"=w259) -> ("error out"=w256:errorcluster)  [unwired: 4 in, 4 out]
              }
            }
            n114 = property class="Str"(reference=w244, "Value"=w247) -> ()  [unwired: 1 in, 2 out]
            n115 = Bundle By Name(cluster=w238, "System Set"=T2 FALSE, "Data OK"=TRUE, "Graph Data"=w237) -> (w236:T12)
          }
          frame #2 {
            n116 = Tick Count (ms)() -> (millisecond timer value=→"End acq":u32)
          }
          frame #3 {
            n117 = local read "Begin acq"() -> (w267:u32)
            n118 = local read "End acq"() -> (w268:u32)
            n119 = Subtract(x=w268, y=w267) -> (x-y=w266:u32)
            n120 = Divide(x=w266, y=u32 1000) -> (x/y=→"Time needed(s)":dbl)
          }
        }
      }
      frame "Load Data" {
        # "Load Data - Loads data from a TDMS file and incorporates it with the existing data according to the user's preference."
        n121 = call "Load Data.vi"("error in (no error)"=w273) -> ("error out"=w279:errorcluster, "New Graph Data"=w277:waveform(dbl)[])  [unwired: 9 in]
        n122 = case shown="No Error" w279 {
          selector: w279 -> [w284 w289]
          tunnel: [w281 w287] -> w275
          tunnel: w277 -> [w283 _]
          tunnel: ["Data loaded." ("Data loaded") "Data not loaded." ("Data not loaded")] -> w278
          tunnel: w276 -> [w282 w287]
          tunnel: [w284 w286] -> w272
          frame No Error {
            n123 = Bundle By Name(cluster=w282, "Graph Data.Data"=w283) -> (w281:T12)
          }
          frame Error {
            n124 = call <vilib>:"Simple Error Handler.vi"("error in (no error)"=w289) -> ("error out"=w286:errorcluster)  [unwired: 4 in, 4 out]
          }
        }
        n125 = Unbundle By Name(w275) -> ("UI References.Status Ref"=w274:refnum<vi>)
        n126 = property class="Str"(reference=w274, "Value"=w278) -> ()  [unwired: 1 in, 2 out]
      }
      frame "Save Data" {
        # "Save Data - Saves the existing measurement data to a TDMS file."
        n127 = Unbundle By Name(w292) -> ("UI References.Status Ref"=w293:refnum<vi>, "Graph Data.Data"=w294:waveform(dbl)[])
        n128 = call "Save Data.vi"("error in (no error)"=w291, "Data"=w294) -> ("error out"=w296:errorcluster)  [unwired: 9 in]
        n129 = case shown="No Error" w296 {
          selector: w296 -> [w298 w302]
          tunnel: ["Data saved." ("Data saved") "Data not saved." ("Data not saved")] -> w295
          tunnel: [w298 w300] -> w290
          frame No Error {
          }
          frame Error {
            n130 = call <vilib>:"Simple Error Handler.vi"("error in (no error)"=w302) -> ("error out"=w300:errorcluster)  [unwired: 4 in, 4 out]
          }
        }
        n131 = property class="Str"(reference=w293, "Value"=w295) -> ()  [unwired: 1 in, 2 out]
      }
      frame "Export Data" {
        # "Export Data - Exports the currently loaded measurement and analysis data to a text file that can be imported into a spreadsheet or other application."
        n132 = Unbundle By Name(w305) -> ("UI References.Status Ref"=w306:refnum<vi>, "Graph Data"=w307:T14)
        n133 = call "Export Data.vi"("error in (no error)"=w304, "Graph Data"=w307) -> ("error out"=w308:errorcluster)  [unwired: 9 in]
        n134 = case shown="No Error" w308 {
          selector: w308 -> [w311 w315]
          tunnel: ["Data exported." ("Data exported") "Data not exported." ("Data not exported")] -> w309
          tunnel: [w311 w313] -> w303
          frame No Error {
          }
          frame Error {
            n135 = call <vilib>:"Simple Error Handler.vi"("error in (no error)"=w315) -> ("error out"=w313:errorcluster)  [unwired: 4 in, 4 out]
          }
        }
        n136 = property class="Str"(reference=w306, "Value"=w309) -> ()  [unwired: 1 in, 2 out]
      }
      frame "Clear Data" {
        # "Clear Data - Clears the data currently in the graph."
        n137 = Bundle By Name(cluster=w318, "Graph Data"=T14 {"Data"=[], "Annotation List"=[], "Cursor List"=[], "Analysis Data"=[]} ("Graph")) -> (w317:T12)
      }
      frame "Analyze" {
        # "#CodeRecommended - Add your own signal analysis here."
        # "Analyze - Analyzes the measurement data."
        n138 = global read "Global ADCarray.vi" "ADC array"() -> (w326:i32[][])
        n139 = call "Analysiswangtest.vi"("error in (no error)"=w325, "ADC array"=w326) -> ("error out"=w324:errorcluster, "Results"=w322:T5)  [unwired: 8 in]
        n140 = Bundle By Name(cluster=w323, "Results"=w322) -> (w321:T12)
      }
      frame "Curve fitting" {
      }
      frame "Copy Graph" {
        # "Copy Graph - Places an image of the graph on the clipboard for pasting into reports or emails."
        n141 = call "Copy Graph to Clipboard.vi"("error in (no error)"=w332, "Graph Data"=w333) -> ("error out"=w331:errorcluster)  [unwired: 9 in]
      }
      frame "Exit" {
        w337 = TRUE  # Stop Loop?
        w338 = State."Exit"  # (Value Not Used)
        # "Exit ----stops execution."
      }
      frame "Load config" {
        n142 = Unbundle By Name(w344) -> ("User Specified"=w346:T17)
        n143 = call "Load Configuration Settings from XML.vi"("error in (no error)"=w341, "User Configuration in"=w346) -> ("error out"=w340:errorcluster, "User Configuration out"=w345:T17)  [unwired: 8 in]
        n144 = Bundle By Name(cluster=w344, "User Specified"=w345, "System Set"=T2 FALSE) -> (w343:T12)
      }
      frame "Save config" {
        # "Save config -  Saves the user's settings to an XML file"
        n145 = Unbundle By Name(w349) -> ("UI References.Status Ref"=w347:refnum<vi>, "User Specified"=w352:T17)
        n146 = call "Save Configuration Settings to XML.vi"("error in (no error)"=w351, "User Configuration"=w352) -> ("error out"=w350:errorcluster)  [unwired: 9 in]
        n147 = property class="Str"(reference=w347, "Value"="Application exit." ("Stopped")) -> ()  [unwired: 1 in, 2 out]
      }
    }
    n148 = Or(x=w5, y=w10) -> (x .or. y?=w9:bool)
  }
  n149 = call <vilib>:"Simple Error Handler.vi"("error in (no error)"=w4) -> ("error out"=w3:errorcluster)  [unwired: 4 in, 4 out]
  n150 = disable-structure shown="RUN_TIME_ENGINE==True" {
    disable-tunnel: w3 -> [_ _]
    frame condition #0 (active) {
    }
    frame condition #1 {
      # "Call Quit LabVIEW if running as a built application."
      n151 = Quit LabVIEW() -> ()  [unwired: 1 in]
    }
  }
